vi "Enable Group Filtering.vi"(0 "Display State In":T2={"Hierarchy"=[], "File/Directory Path"=path "", "Relative File Paths"=[], "Hide Undefined Channels"=FALSE, "Static File Structure"=FALSE, "Filtering"={"Filtered Groups"=[], "Group Filter Mode"=enum."Exclude", "Group Filter Regex?"=FALSE, "Filtered Channels"=[], "Channel Filter Mode"=enum."Exclude", "Channel Filter Regex?"=FALSE, "Filter Time Start"=timestamp(0 s since 1904-01-01), "Filter Time End"=timestamp(0 s since 1904-01-01), "Time Filter Mode"=enum."Include", "Time Filter Enabled"=FALSE}, "File Contents Tree"=refnum, "Properties Table"=refnum, "Loading Indicator"=refnum}, 1 "Use Regular Expressions?":bool, 5 "Filter Mode":T1, 7 "Group Names":string[](array[string]), 9 "Container State":T4, 11 "error in (no error)":errorcluster) -> (4 "Display State Out":T2={"Hierarchy"=[], "File/Directory Path"=path "", "Relative File Paths"=[], "Hide Undefined Channels"=FALSE, "Static File Structure"=FALSE, "Filtering"={"Filtered Groups"=[], "Group Filter Mode"=enum."Exclude", "Group Filter Regex?"=FALSE, "Filtered Channels"=[], "Channel Filter Mode"=enum."Exclude", "Channel Filter Regex?"=FALSE, "Filter Time Start"=timestamp(0 s since 1904-01-01), "Filter Time End"=timestamp(0 s since 1904-01-01), "Time Filter Mode"=enum."Include", "Time Filter Enabled"=FALSE}, "File Contents Tree"=refnum, "Properties Table"=refnum, "Loading Indicator"=refnum}, 15 "error out":errorcluster)   [LabVIEW 2017, in "XTree.xctl"]
doc: "Enables group filtering with the specified settings. The Group Names input supports regular expressions. Tree will need to be repopulated to reflect new settings."
uses:
  <vilib>/addons/_NIFileIO/XTree/XTree.xctl
  <vilib>/_xctls/Container State.ctl
  <vilib>/addons/_NIFileIO/XTree/State.ctl
  <vilib>/addons/_NIFileIO/XTree/Controls/Filter Settings.ctl
  <vilib>/addons/_NIFileIO/XTree/Controls/Filter Mode.ctl
  <vilib>/_xctls/XControlSupport.lvlib
panel:
  # "Add Controls & Indicators that form the parameters of the method here. Hook them to the connector pane. Do not delete the controls & indicators that are already hooked to the connector pane.\n \nTo setup the parameters  for this method, right click on this item in the Project Tree & select \"Configure Method...\"."
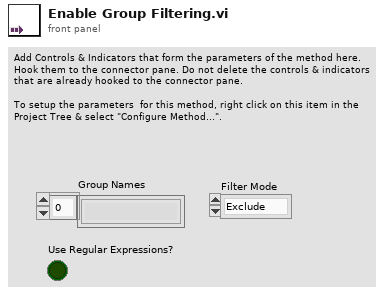
[diagram p1: front panel]
types:
  T1 = typedef "XTree.xctl/Filter Mode.ctl" = enum16{"Exclude", "Include"}
  T2 = typedef "XTree.xctl/State.ctl" = cluster{"Hierarchy":string[], "File/Directory Path":path, "Relative File Paths":string[], "Hide Undefined Channels":bool, "Static File Structure":bool, "Filtering":T3, "File Contents Tree":refnum<vi>, "Properties Table":refnum<vi>, "Loading Indicator":refnum<vi>}
  T3 = typedef "XTree.xctl/Filter Settings.ctl" = cluster{"Filtered Groups":string[], "Group Filter Mode":T1, "Group Filter Regex?":bool, "Filtered Channels":string[], "Channel Filter Mode":T1, "Channel Filter Regex?":bool, "Filter Time Start":timestamp, "Filter Time End":timestamp, "Time Filter Mode":T1, "Time Filter Enabled":bool}
  T4 = typedef "XControlSupport.lvlib/Container State.ctl" = cluster{"Indicator?":bool, "Run Mode?":bool, " Refnum":refnum<vi>}
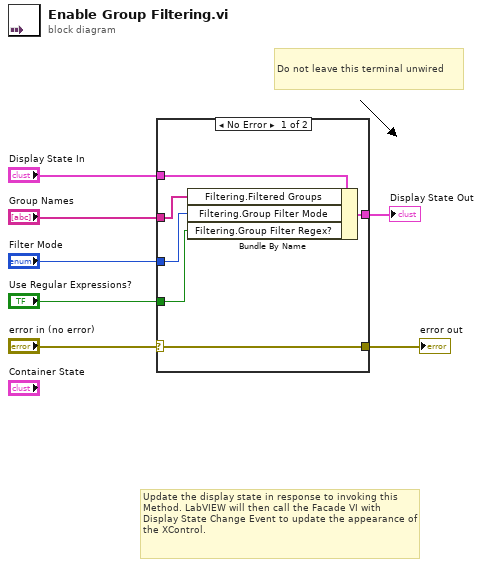
[diagram p0: block diagram]
diagram:
  # "Do not leave this terminal unwired"
  # "Update the display state in response to invoking this Method. LabVIEW will then call the Facade VI with Display State Change Event to update the appearance of the XControl."
  n1 = case shown="No Error" "error in (no error)" {
    selector: "error in (no error)" -> [w11 w14]
    tunnel: "Display State In" -> [w13 w15]
    tunnel: [w12 w15] -> w6
    tunnel: [w11 w14] -> w4
    tunnel: "Group Names" -> [w10 _]
    tunnel: "Filter Mode" -> [w9 _]
    tunnel: "Use Regular Expressions?" -> [w8 _]
    frame No Error {
      n2 = Bundle By Name(cluster=w13, "Filtering.Filtered Groups"=w10, "Filtering.Group Filter Mode"=w9, "Filtering.Group Filter Regex?"=w8) -> (w12:T2)
    }
    frame Error {
    }
  }
  "Display State Out" <- w6
  "error out" <- w4
